vi "SCLN_GlobalQueues.vi"(6 "Write QueueID":refnum<queue>, 7 "Element":i32, 8 "Operation":i32 min=0 max=1, 9 "Number of Elements":i32=10) -> (0 "Queue Array Out":refnum<queue>[](array[refnum]), 3 "Read QueueID":refnum<queue>)   [LabVIEW 2015]
doc: "Handle Queue Globals Style II.\nThe globals are maintained in an uninitialized \nshift register, as an array of queues.\nTherefore, It is mandatory to initialize each element \nof the array in a sequential way.\n\nINPUTS:\n Operation: TRUE = WRITE, FALSE = READ\n Element: Element of the array to write or read\n Write Value: Queue value to store\nOUTPUTS:\n Read Value: Queue value retrieved\n Queue Array Out: The entire array of queues"
panel:
  # "1 = WRITE  WRITE"
  # "0 = READ"
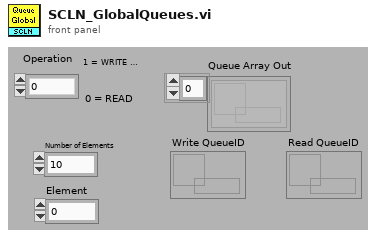
[diagram p1: front panel]
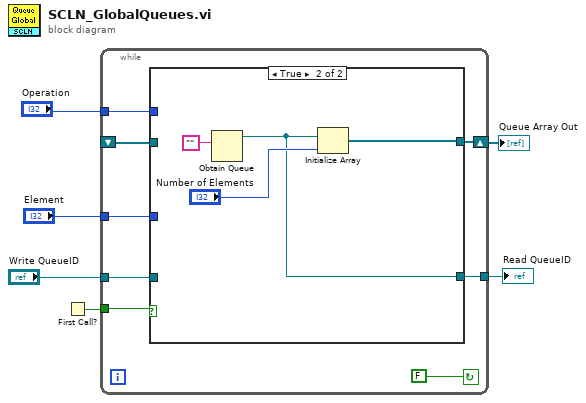
[diagram p0: block diagram]
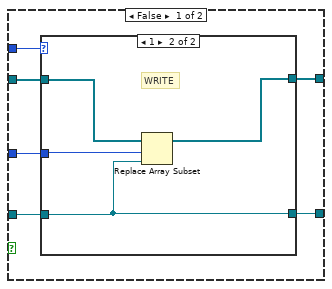
[diagram p2: hidden frame]
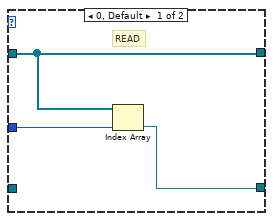
[diagram p3: hidden frame]
diagram:
  n1 = First Call?() -> (First Call?: T/F=w5:bool)
  n2 = while {
    tunnel: "Operation" -> [w13]
    shift-right: [w12] -> w4
    shift-left: _ -> [w11]
    tunnel: "Element" -> [w10]
    tunnel: "Write QueueID" -> [w9]
    tunnel: [w8] -> w1
    tunnel: w5 -> [w7]
    stop <- FALSE continue-if-true
    n3 = case shown="True" w7 {
      tunnel: w13 -> [w20 _]
      tunnel: [w19 w31] -> w12
      tunnel: w11 -> [w18 _]
      tunnel: w10 -> [w17 _]
      tunnel: w9 -> [w16 _]
      tunnel: [w15 w28] -> w8
      frame False {
        n4 = case shown="1" w20 {
          tunnel: [w21 w27] -> w19
          tunnel: w18 -> [w21 w26]
          tunnel: w17 -> [w23 w25]
          tunnel: w16 -> [_ w24]
          tunnel: [w22 w24] -> w15
          frame 0, Default {
            # "READ"
            n5 = Index Array(array=w21, index=w23) -> (element=w22:refnum<queue>)
          }
          frame 1 {
            # "WRITE"
            n6 = Replace Array Subset(array=w26, new element=w24, index=w25) -> (w27:refnum<queue>[])
          }
        }
      }
      frame True {
        n7 = Obtain Queue(element data type="") -> (queue out=w28:refnum<queue>)  [unwired: 4 in, 2 out]
        n8 = Initialize Array(w28, "Number of Elements") -> (w31:refnum<queue>[])
      }
    }
  }
  "Queue Array Out" <- w4
  "Read QueueID" <- w1
